vi "ZDataVIS_Configure_Intensity_Plot.vi"(4 "swap x and y?":bool=TRUE, 5 "autoName":bool, 6 "XYZ Variable Selection":T1, 7 "Scan Name":string[](array[string]), 8 "error in (no error)":errorcluster, 9 "Y Offset and Multiplier":T2, 10 "X Offset and Multiplier":T2, 11 "IntensityGraph in":refnum<vi>) -> (0 "error out":errorcluster)   [LabVIEW 2016]
uses:
  <vilib>/Utility/miscctls.llb/LVOffsetAndMultiplierTypeDef.ctl
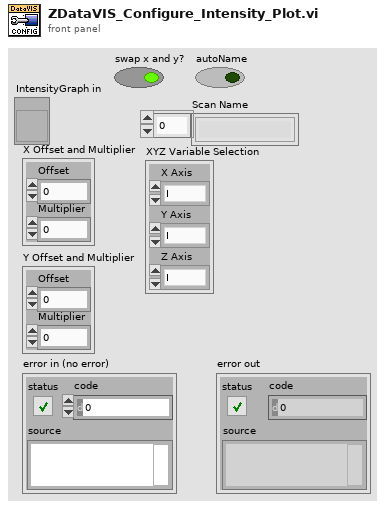
[diagram p1: front panel]
types:
  T1 = cluster{"X Axis":enum16{"I", "Vsd", "V4T", "dI/dV 2T", "dV/dI 2T", "dV/dI 4T", "dI/dV 4T"}, "Y Axis":enum16{"I", "Vsd", "V4T", "dI/dV 2T", "dV/dI 2T", "dV/dI 4T", "dI/dV 4T"}, "Z Axis":enum16{"I", "Vsd", "V4T", "dI/dV 2T", "dV/dI 2T", "dV/dI 4T", "dI/dV 4T"}}
  T2 = typedef "LVOffsetAndMultiplierTypeDef.ctl" = cluster{"Offset":dbl, "Multiplier":dbl}
  T3 = enum16{"I", "Vsd", "V4T", "dI/dV 2T", "dV/dI 2T", "dV/dI 4T", "dI/dV 4T"}
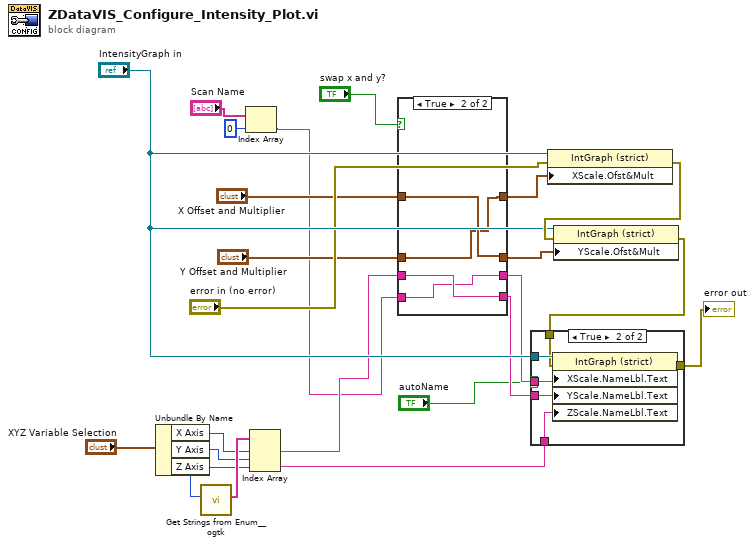
[diagram p0: block diagram]
diagram:
  n1 = Unbundle By Name("XYZ Variable Selection") -> ("X Axis"=w19:T3, "Y Axis"=w18:T3, "Z Axis"=w17:T3)
  n2 = call <userlib>:"Get Strings from Enum__ogtk.vi"("Enum"=w17) -> ("Enum Strings"=w20:string[])  [unwired: 7 in, 3 out]
  n3 = Index Array(array="Scan Name", index=0) -> (element=w5:string)
  n4 = Index Array(array=w20, index #1=w19, index #2=w18, index #3=w17) -> (element #1=w6:string, element #3=w16:string)  [unwired: 1 out]
  n5 = case shown="True" "swap x and y?" {
    tunnel: "X Offset and Multiplier" -> [w27 w31]
    tunnel: [w27 w30] -> w9
    tunnel: "Y Offset and Multiplier" -> [w26 w30]
    tunnel: [w26 w31] -> w7
    tunnel: w6 -> [w25 w29]
    tunnel: w5 -> [w24 w28]
    tunnel: [w25 w28] -> w4
    tunnel: [w24 w29] -> w3
    frame False {
    }
    frame True {
    }
  }
  n6 = property class="IntGraph (strict)"(reference="IntensityGraph in", error in="error in (no error)", "XScale.Ofst&Mult"=w9) -> (error out=w23:errorcluster)  [unwired: 1 out]
  n7 = property class="IntGraph (strict)"(reference="IntensityGraph in", error in=w23, "YScale.Ofst&Mult"=w7) -> (error out=w13:errorcluster)  [unwired: 1 out]
  n8 = case shown="True" "autoName" {
    tunnel: "IntensityGraph in" -> [_ w38]
    tunnel: w16 -> [_ w37]
    tunnel: [w32 w36] -> w14
    tunnel: w13 -> [w32 w35]
    tunnel: w4 -> [_ w34]
    tunnel: w3 -> [_ w33]
    frame False {
    }
    frame True {
      n9 = property class="IntGraph (strict)"(reference=w38, error in=w35, "XScale.NameLbl.Text"=w34, "YScale.NameLbl.Text"=w33, "ZScale.NameLbl.Text"=w37) -> (error out=w36:errorcluster)  [unwired: 1 out]
    }
  }
  "error out" <- w14
